vi "dhtSensor.vi"() -> ()   [LabVIEW 2018]
uses:
  <vilib>/rvi/Emulation/niFpgaGetClockAttributes.vi
  <vilib>/rvi/Emulation/niFpgaSctlEmulationGetInTimedLoop.vi
  <vilib>/rvi/Emulation/niFpgaEmulationReportErrorSimple.vi
  <vilib>/rvi/eio/common/nirviEmuTemplateMethod_errors.vi
  <vilib>/rvi/Emulation/niFpgaCriticalErrorInLSC.vi
  <vilib>/eio/EIOMethodNode/EIOMethodNode.xnode
  <vilib>/eio/EIONode/EIONode.xnode
panel:
  out "Array":i16[](array[numeric])
  out "Read Time":i16
  out "Temperature":i16(slide) scale=0.0..100.0
  out "Humidity":i16
  in  "stop":bool
  in  "11 - 22":bool
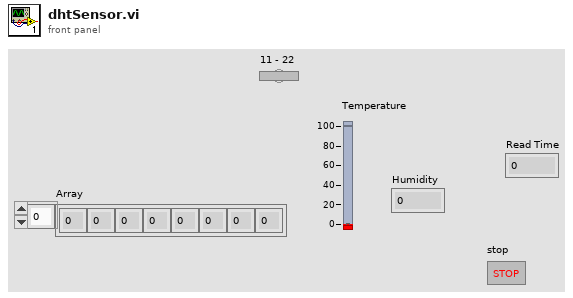
[diagram p1: front panel]
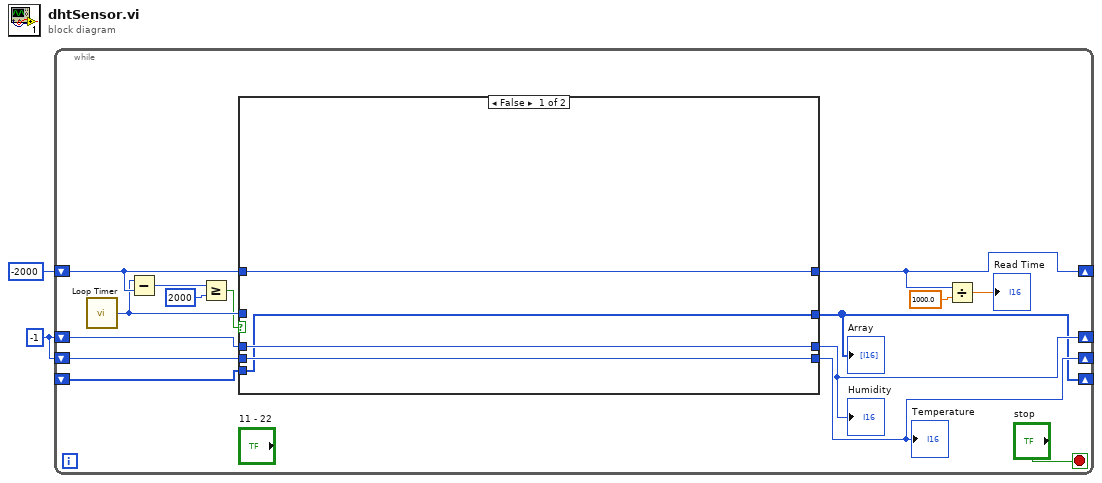
[diagram p0: block diagram]
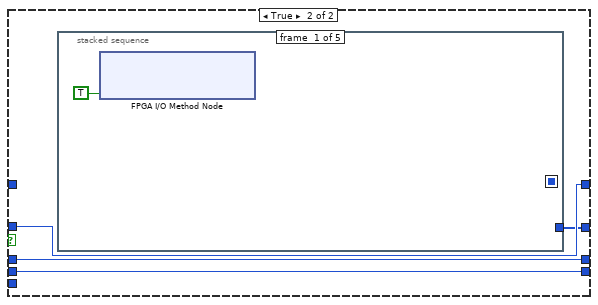
[diagram p2: hidden frame]
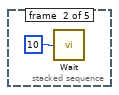
[diagram p3: hidden frame]
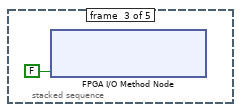
[diagram p4: hidden frame]
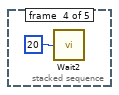
[diagram p5: hidden frame]
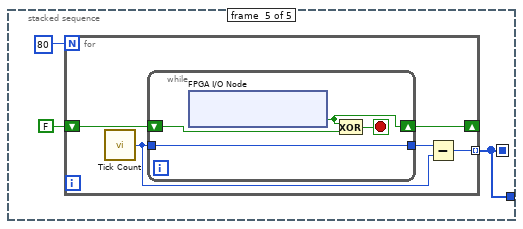
[diagram p6: hidden frame]
diagram:
  w1 = i16 -1
  n1 = while {
    shift-right: [w10] -> _
    shift-left: i16 -2000 -> [w12]
    shift-right: [w13] -> _
    shift-left: w1 -> [w15]
    shift-right: [w14] -> _
    shift-left: w1 -> [w16]
    shift-right: [w6] -> _
    shift-left: _ -> [w7]
    stop <- "stop" stop-if-true
    n2 = call "Loop Timer"() -> ("Tick Count(mSec)"=w11:u32)  [unwired: 1 in]
    n3 = Subtract(x=w11, y=w12) -> (x-y=w5:u32)
    n4 = Greater Or Equal?(x=w5, y=i16 2000) -> (x >= y?=w4:bool)
    n5 = case shown="False" w4 {
      tunnel: [w21 w24] -> w14
      tunnel: [w20 w23] -> w13
      tunnel: w16 -> [w21 w24]
      tunnel: w15 -> [w20 w23]
      tunnel: [w19 w25] -> w10
      tunnel: w12 -> [w19 _]
      tunnel: w11 -> [_ w25]
      tunnel: [w18 w22] -> w6
      tunnel: w7 -> [w18 _]
      frame False {
      }
      frame True {
        n6 = stacked-sequence {
          seq-local: [_ _ _ _ w30] -> [_ _ _ _ _]
          tunnel: [_ _ _ _ w30] -> w22
          frame #0 {
            n7 = xnode "FPGA I/O Method Node"("Data"=TRUE) -> ()  [unwired: 1 in, 1 out]
          }
          frame #1 {
            n8 = call "Wait"("Count(mSec)"=i16 10) -> ()  [unwired: 1 out]
          }
          frame #2 {
            n9 = xnode "FPGA I/O Method Node"("Data"=FALSE) -> ()  [unwired: 1 in, 1 out]
          }
          frame #3 {
            n10 = call "Wait2"("Count(mSec)"=i16 20) -> ()  [unwired: 1 out]
          }
          frame #4 {
            n11 = for {
              N: i16 80 -> [_]
              shift-right: [w37] -> _
              shift-left: FALSE -> [w36]
              tunnel: [w33] -> w30 mode=indexing
              n12 = call "Tick Count"() -> ("Tick Count(uSec)"=w34:u32)
              n13 = while {
                tunnel: [w38] -> w35
                tunnel: w34 -> [w38]
                shift-right: [w39] -> w37
                shift-left: w36 -> [w41]
                stop <- w40 stop-if-true
                n14 = xnode "FPGA I/O Node"() -> ("ConnectorA/DIO3"=w39:bool)  [unwired: 1 in, 1 out]
                n15 = Exclusive Or(1:w41, 2:w39) -> (0:w40:bool)
              }
              n16 = Subtract(x=w35, y=w34) -> (x-y=w33:u32)
            }
          }
        }
      }
    }
    "Humidity" <- w14
    "Temperature" <- w13
    "Array" <- w6
    n17 = Divide(x=w10, y=sgl 1000.0) -> (x/y=→"Read Time":sgl)
  }
